vi "stop.vi"(8 "error in (no error)":errorcluster, 11 "identifier":string) -> (0 "error out":errorcluster, 3 "function return":u32)   [LabVIEW 2015, in "XGL_DPP.lvlib"]
doc: "EXTERN DECLSPEC unsigned int CALL_CONV stop(const char* identifier);"
uses:
  XGL_DPP.lvlib
  XGL_DPP.dll
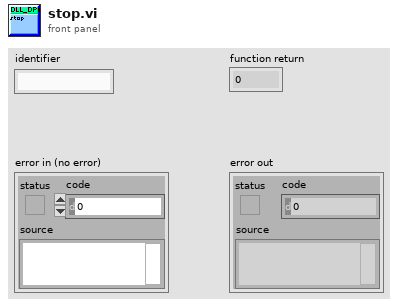
[diagram p1: front panel]
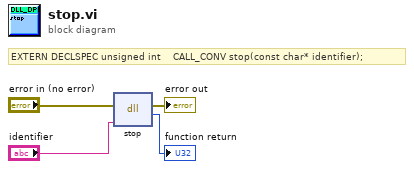
[diagram p0: block diagram]
diagram:
  # "EXTERN DECLSPEC unsigned int    CALL_CONV stop(const char* identifier);"
  n1 = dll-call lib="D:/Users/XRF/Desktop/Dante_acquire4/libs/Dante/XGL_DPP.*" fn="stop"(error in="error in (no error)", "identifier"="identifier") -> (error out=→"error out":errorcluster, "return type"=→"function return":u32)  [unwired: 3 in, 1 out]
